vi "Inst.TC.DoSomething.vi"(8 "error in (no error)":errorcluster, 10 "Data":variant, 11 "Inst.TC in":refnum<class "Inst.TC.lvclass">) -> (0 "error out":errorcluster, 2 "Data out":variant, 3 "Inst.TC out":refnum<class "Inst.TC.lvclass">)   [LabVIEW 2019, in "Inst.TC.lvclass"]
uses:
  Inst.TC.lvclass
  fdab1b40-c942-4d42-9f74-5965e28da6e4.vi
  <vilib>/JDP Science/JSONtext/JSON text to Variant.vi
  <vilib>/JDP Science/JSONtext/LVClass Serializer/JSONtext LVClass Serializer.lvclass
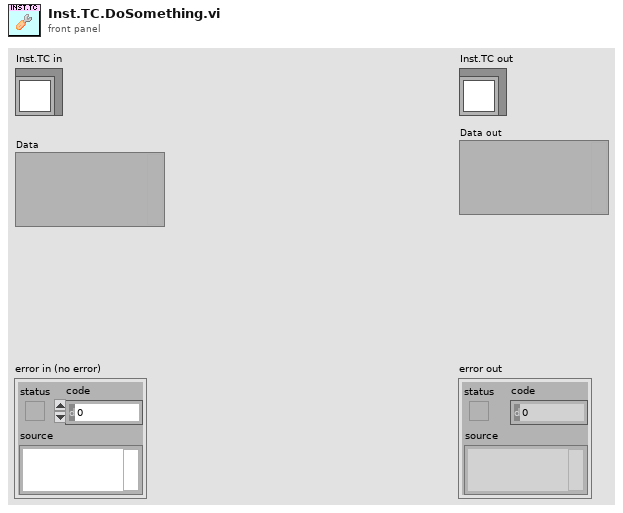
[diagram p1: front panel]
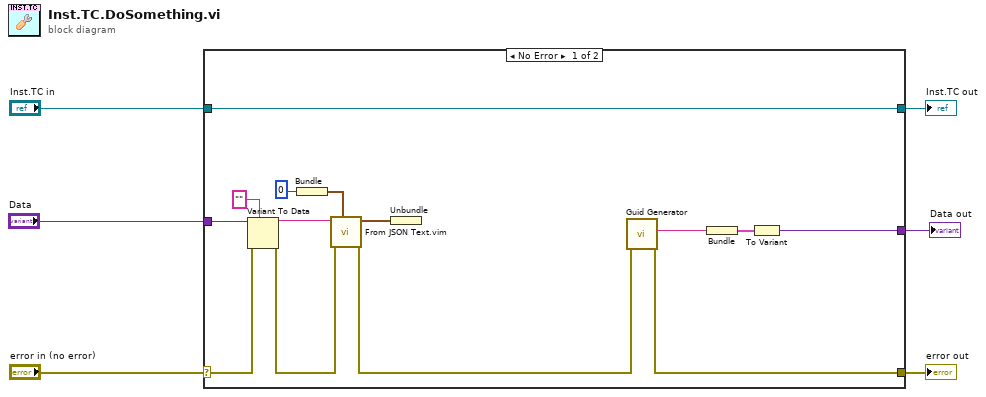
[diagram p0: block diagram]
diagram:
  n1 = case shown="No Error" "error in (no error)" {
    selector: "error in (no error)" -> [w18 w22]
    tunnel: [w11 w22] -> w5
    tunnel: [w8 w21] -> w3
    tunnel: "Inst.TC in" -> [w8 w21]
    tunnel: "Data" -> [w20 _]
    tunnel: [w10 _] -> w1
    frame No Error {
      n2 = Variant To Data(error in=w18, type="", Variant=w20) -> (data=w17:string, error out=w16:errorcluster)
      n3 = Bundle("bytes to read"=0) -> (w15:cluster{"bytes to read":i32})  [unwired: 1 in]
      n4 = call "From JSON Text.vim"("Data Type and Default Value"=w15, "error in (no error)"=w16, "JSON"=w17) -> ("error out"=w7:errorcluster, "Data out"=w14:cluster{"bytes to read":i32})  [unwired: 7 in]
      n5 = Unbundle(w14) -> ()  [unwired: 1 out]
      n6 = call <vilib>:"Guid Generator.vi"("error in (no error)"=w7) -> ("error out"=w11:errorcluster, "GUID"=w12:string)  [unwired: 9 in]
      n7 = Bundle("GUID"=w12) -> (w9:cluster{"GUID":string})  [unwired: 1 in]
      n8 = To Variant(anything=w9) -> (Variant=w10:variant)
    }
    frame Error {
    }
  }
  "error out" <- w5
  "Inst.TC out" <- w3
  "Data out" <- w1
